vi "Get Object by Type.vi"(8 "error in (no error)":errorcluster, 10 "Type":refnum<class "Analyze Results Base.lvclass">, 11 "Analyze Compound Results Base in":refnum<class "Analyze Compound Results Base.lvclass">) -> (0 "error out":errorcluster, 1 "found?":bool, 2 "Result Obj":refnum<class "Analyze Results Base.lvclass">, 3 "Analyze Compound Results Base out":refnum<class "Analyze Compound Results Base.lvclass">)   [LabVIEW 2014, in "Analyze Compound Results Base.lvclass"]
uses:
  Analyze Compound Results Base.lvclass
  Results Base/Analyze Results Base.lvclass
  Analyze Compound Results Base.lvclass/Analyze Compound Results Base.ctl
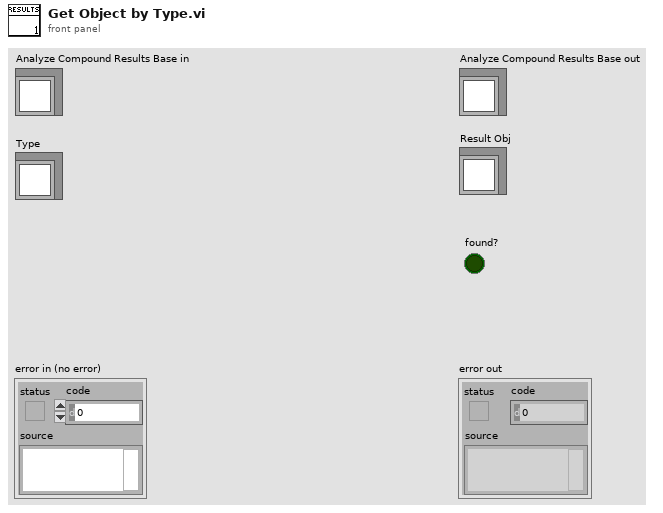
[diagram p1: front panel]
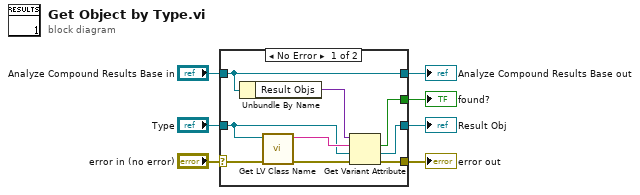
[diagram p0: block diagram]
diagram:
  n1 = case shown="No Error" "error in (no error)" {
    selector: "error in (no error)" -> [w10 w19]
    tunnel: [w9 w19] -> w6
    tunnel: [w16 w18] -> w4
    tunnel: "Analyze Compound Results Base in" -> [w16 w18]
    tunnel: "Type" -> [w8 w17]
    tunnel: [w12 w17] -> w2
    tunnel: [w11 _] -> w1
    frame No Error {
      n2 = Unbundle By Name(w16) -> ("Result Objs"=w15:variant)
      n3 = call <vilib>:"Get LV Class Name.vi"("error in (no error)"=w10, "object"=w8) -> ("error out"=w13:errorcluster, "class name"=w14:string)  [unwired: 8 in]
      n4 = Get Variant Attribute(Variant=w15, name=w14, default value (empty Variant)=w8, error in=w13) -> (found=w11:bool, value=w12:refnum<class "Analyze Results Base.lvclass">, error out=w9:errorcluster)  [unwired: 1 out]
    }
    frame Error {
    }
  }
  "error out" <- w6
  "Analyze Compound Results Base out" <- w4
  "Result Obj" <- w2
  "found?" <- w1
